vi "Vision_Right_R12.vi"() -> ()   [LabVIEW 2015]
uses:
  <vilib>/vision/Pattern Matching.llb/IMAQ Curve Parameters.ctl
  <vilib>/vision/Pattern Matching.llb/IMAQ Match Range Setting.ctl
panel:
  out "Tracking Info":T1
  out "dT":u32
  out "Avg Scale":dbl=50.23627395629883
  out "Avg Score":dbl=800.1138671875
  out "Current Search Settings":T4={"Curve Parameters"={"Extraction Mode"=1, "Edge Threshold"=150, "Edge Filter Size"=0, "Min Length"=25, "Row Search Step Size"=15, "Col Search Step Size"=15, "Max Endpoint Gap"=2, "Closed"=TRUE, "Subpixel"=TRUE}, "Match Mode"={"Rotation"=TRUE, "Scale"=TRUE, "Occlusion"=TRUE, "Reserved"=FALSE, "Reserved"=FALSE, "Reserved"=FALSE}, "Range Settings"=[{"Match Constraints"=0, "Min"=-5.0, "Max"=5.0}, {"Match Constraints"=1, "Min"=45.23627395629883, "Max"=55.23627395629883}, {"Match Constraints"=2, "Min"=0.0, "Max"=25.0}], "Number of Matches"=1, "Minimum Match Score"=700.1139, "SubPixel Accuracy"=TRUE, "Adv. Geometric Match Options 2"=[{"Setup Data Item"=20, "Item Value"=0.0}, {"Setup Data Item"=22, "Item Value"=1.0}]} {"Curve Parameters"."Extraction Mode" items=["Normal", "Uniform Regions"]; "Curve Parameters"."Edge Filter Size" items=["Fine", "Normal", "Contour Tracing"]; "Curve Parameters"."Max Endpoint Gap" min=0; "Curve Parameters"."Col Search Step Size" min=1 max=255 step=1; "Curve Parameters"."Row Search Step Size" min=1 max=255 step=1; "Curve Parameters"."Min Length" min=0; "Curve Parameters"."Edge Threshold" min=1 max=350 step=1; "Range Settings"."Max" format="%.2f"; "Range Settings"."Min" format="%.2f"; "Range Settings"."Match Constraints" items=["Rotation Angle (degrees)", "Scale Factor (%)", "Occlusion (%)"]}
  out "Valid Scale History":dbl[](array[numeric])=[50.547454833984375, 50.07851791381836, 50.25061798095703, 50.25061798095703, 50.054161071777344, 50.02944564819336, 50.078575134277344, 50.081233978271484, 50.078975677490234, 50.078575134277344, 50.07851791381836, 50.6029052734375, 50.602447509765625, 50.602447509765625, 50.58179473876953, 51.42407989501953, 50.560218811035156, 51.42409896850586, 0.0, 50.602447509765625] format="%#_13g"
  out "Valid Score History":dbl[](array[numeric])=[802.5203247070312, 804.2725830078125, 794.4934692382812, 794.4934692382812, 804.7894897460938, 809.00341796875, 804.2725830078125, 805.539794921875, 804.2725830078125, 803.1467895507812, 804.2725830078125, 777.2046508789062, 774.6702270507812, 774.6702270507812, 777.9379272460938, 790.3563232421875, 777.9379272460938, 790.3563232421875, 0.0, 777.2046508789062] format="%#_13g"
  out "Valid Beacon History - in":bool[](array[boolean])=[TRUE, TRUE, TRUE, TRUE, TRUE, TRUE, TRUE, TRUE, TRUE, TRUE, TRUE, TRUE, TRUE, TRUE, TRUE, TRUE, TRUE, TRUE, FALSE, TRUE]
  out "Startup Flag":bool
  out "Current Tempalte State":T5(ring)=enum."Short Range"
  out "Lock Status":bool=TRUE
  out "Y Coordinates":sgl[](array[numeric])=[153.02994, 149.48933, 150.4864, 150.33003, 0.0]
  out "X Coordinates":sgl[](array[numeric])=[91.3685, 123.99656, 161.27843, 197.4523, 0.0]
  out "Beacons Found":bool[](array[boolean])=[TRUE, TRUE, TRUE, TRUE, FALSE]
  out "Right Image out":T6(plugin-control)
  in  "Initial State":T5(ring)=enum."Short Range"
  in  "History Size":i32=20
  in  "INITIAL Search Settings":T4={"Curve Parameters"={"Extraction Mode"=1, "Edge Threshold"=150, "Edge Filter Size"=0, "Min Length"=25, "Row Search Step Size"=15, "Col Search Step Size"=15, "Max Endpoint Gap"=2, "Closed"=TRUE, "Subpixel"=TRUE}, "Match Mode"={"Rotation"=TRUE, "Scale"=TRUE, "Occlusion"=TRUE, "Reserved"=FALSE, "Reserved"=FALSE, "Reserved"=FALSE}, "Range Settings"=[{"Match Constraints"=0, "Min"=-5.0, "Max"=5.0}, {"Match Constraints"=1, "Min"=20.0, "Max"=60.0}, {"Match Constraints"=2, "Min"=0.0, "Max"=25.0}], "Number of Matches"=1, "Minimum Match Score"=750.0, "SubPixel Accuracy"=TRUE, "Adv. Geometric Match Options 2"=[{"Setup Data Item"=20, "Item Value"=0.0}, {"Setup Data Item"=22, "Item Value"=1.0}]} {"Curve Parameters"."Extraction Mode" items=["Normal", "Uniform Regions"]; "Curve Parameters"."Edge Filter Size" items=["Fine", "Normal", "Contour Tracing"]; "Curve Parameters"."Max Endpoint Gap" min=0; "Curve Parameters"."Col Search Step Size" min=1 max=255 step=1; "Curve Parameters"."Row Search Step Size" min=1 max=255 step=1; "Curve Parameters"."Min Length" min=0; "Curve Parameters"."Edge Threshold" min=1 max=350 step=1; "Range Settings"."Max" format="%.2f"; "Range Settings"."Min" format="%.2f"; "Range Settings"."Match Constraints" items=["Rotation Angle (degrees)", "Scale Factor (%)", "Occlusion (%)"]; "Adv. Geometric Match Options 2"."Setup Data Item" items=["Curve Extraction Mode", "Curve Edge Threshold", "Curve Edge Filter Size", "Min Curve Length", "Curve Row Search Step Size", "Curve Col Search Step Size", "Curve Max Endpoint Gap", "Extract Closed Curves", "Enable Subpixel Curve Extraction", "Enable Correlation Score", "Enable Subpixel Accuracy", "Subpixel Iterations", "Subpixel Tolerance", "Initial Match List Length", "Enable Target Template Curve Score", "Min Match Separation Distance", "Min Match Separation Angle", "Min Match Separation Scale", "Max Match Overlap", "Enable Coarse Result", "Enable Calibration Support", "Enable Contrast Reversal", "Search Strategy", "Refinement Match Factor", "Subpixel Match Factor"]}
  # "Range"
  # "Range"
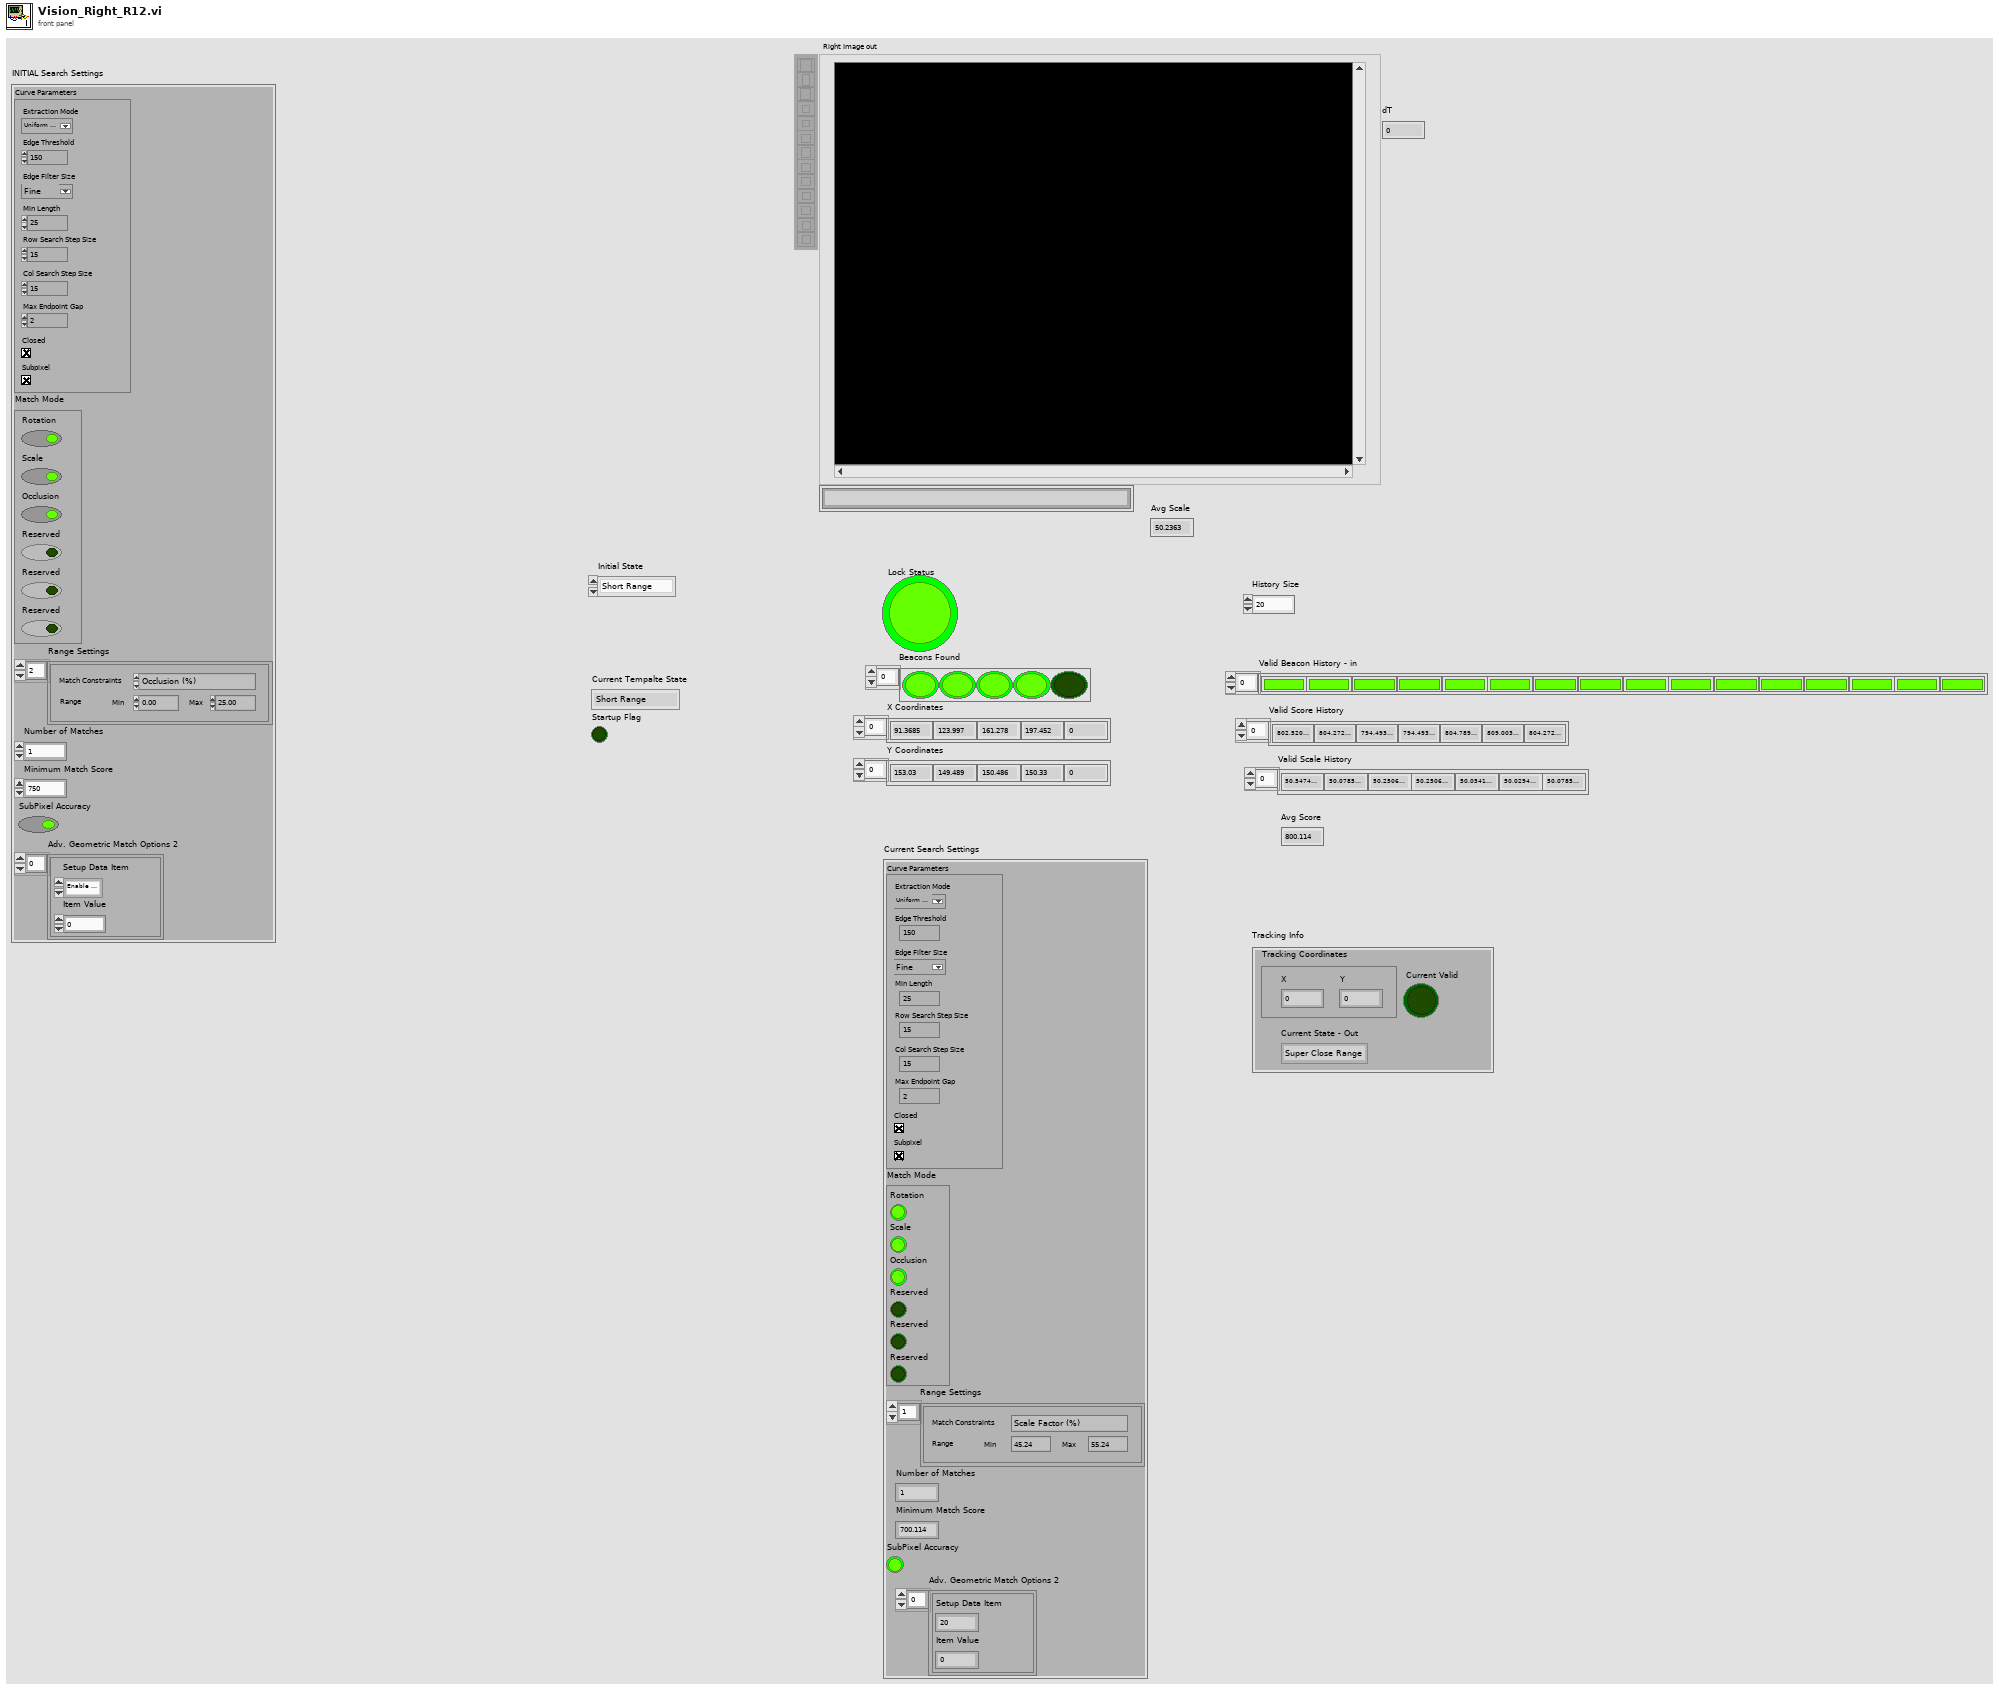
[diagram p1: front panel]
types:
  T1 = cluster{"Tracking Coordinates":cluster{"X":dbl, "Y":dbl}, "Current Valid":bool, "Current State - Out":enum16{"Super Close Range", "Short Range", "Long Range"}}
  T2 = typedef "IMAQ Curve Parameters.ctl" = cluster{"Extraction Mode":u32, "Edge Threshold":i32, "Edge Filter Size":u32, "Min Length":i32, "Row Search Step Size":i32, "Col Search Step Size":i32, "Max Endpoint Gap":i32, "Closed":bool, "Subpixel":bool}
  T3 = typedef "IMAQ Match Range Setting.ctl" = cluster{"Match Constraints":u32, "Min":dbl, "Max":dbl}
  T4 = cluster{"Curve Parameters":T2, "Match Mode":cluster{"Rotation":bool, "Scale":bool, "Occlusion":bool, "Reserved":bool, "Reserved":bool, "Reserved":bool}, "Range Settings":T3[], "Number of Matches":i32, "Minimum Match Score":sgl, "SubPixel Accuracy":bool, "Adv. Geometric Match Options 2":cluster{"Setup Data Item":u16, "Item Value":dbl}[]}
  T5 = enum16{"Super Close Range", "Short Range", "Long Range"}
  T6 = typedef "IMAQ Image.ctl" = refnum<image>
  T7 = typedef "Image Type" = u32
  T8 = typedef "ROI Descriptor" = cluster{"Global Rectangle":i32[], "Contours":cluster{"ID":enum32{"External", "Internal"}, "Type":u32, "Coordinates":i32[]}[]}
  T9 = cluster{"Valid Beacon History\nOut":bool[], "Valid Score History\nOut":dbl[], "Valid Scale History\nOut":dbl[]}
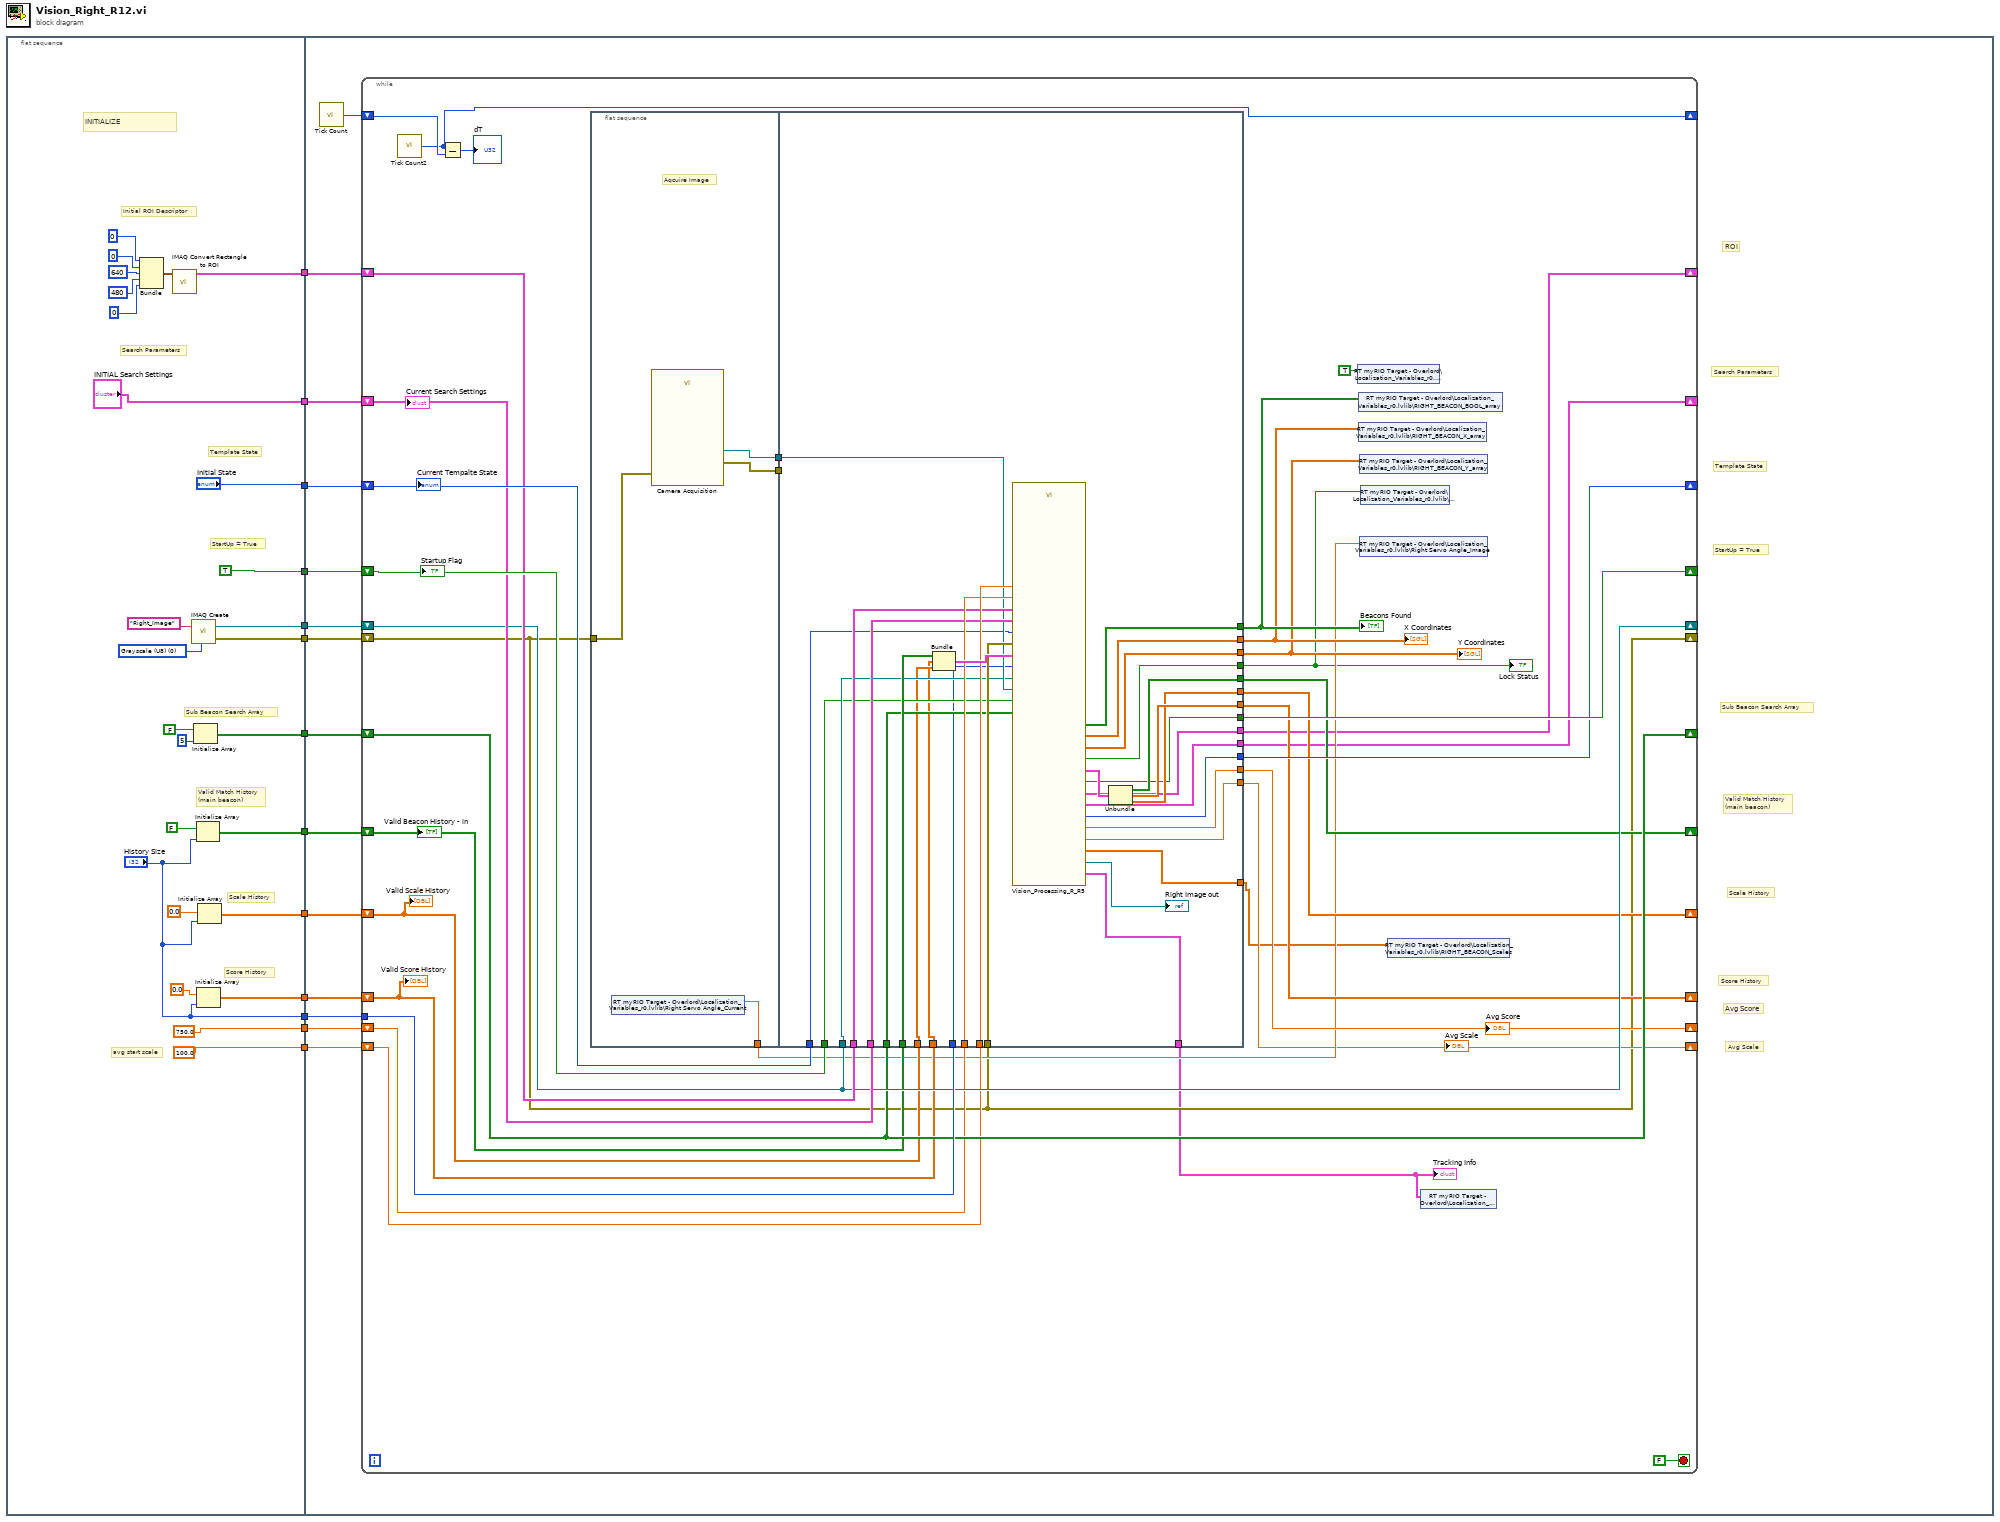
[diagram p0: block diagram]
diagram:
  n1 = flat-sequence {
    tunnel: [w26] -> w13
    tunnel: ["INITIAL Search Settings"] -> w12
    tunnel: ["Initial State"] -> w11
    tunnel: [TRUE] -> w10
    tunnel: [w23] -> w9
    tunnel: [w22] -> w8
    tunnel: [w21] -> w7
    tunnel: [w20] -> w6
    tunnel: [w19] -> w5
    tunnel: [w18] -> w4
    tunnel: ["History Size"] -> w3
    tunnel: [750.0] -> w2
    tunnel: [100.0] -> w1
    tunnel: w13 -> [w53]
    tunnel: w12 -> [w52]
    tunnel: w11 -> [w51]
    tunnel: w10 -> [w50]
    tunnel: w9 -> [w45]
    tunnel: w8 -> [w44]
    tunnel: w7 -> [w49]
    tunnel: w6 -> [w48]
    tunnel: w5 -> [w47]
    tunnel: w4 -> [w46]
    tunnel: w3 -> [w43]
    tunnel: w2 -> [w42]
    tunnel: w1 -> [w41]
    frame #0 {
      w33 = T7 0 items=["Grayscale (U8)", "Grayscale (I16)", "Grayscale (SGL)", "Complex (CSG)", "RGB (U32)", "HSL (U32)", "RGB (U64)", "Grayscale (U16)"] ("Image Type")
      # "avg start scale"
      # "Score History"
      # "Scale History"
      # "Valid Match History\n(main beacon)"
      # "Sub Beacon Search Array"
      # "Template State"
      # "Search Parameters"
      # "StartUp = True"
      # "Initial ROI Descriptor"
      # "INITIALIZE"
      n2 = Bundle(0, 0, 640, 480, 0) -> (w32:cluster{i32, i32, i32, i32, i32})  [unwired: 1 in]
      n3 = call "IMAQ Convert Rectangle to ROI"("Rectangle"=w32) -> ("ROI Descriptor"=w26:T8)  [unwired: 8 in, 1 out]
      n4 = call "IMAQ Create"("Image Name"="Right_Image", "Image Type"=w33) -> ("New Image"=w23:T6, "error out"=w22:errorcluster)  [unwired: 3 in]
      n5 = Initialize Array(FALSE, 5 ("dimension size")) -> (w21:bool[])
      n6 = Initialize Array(FALSE, "History Size") -> (w20:bool[])
      n7 = Initialize Array(0.0, "History Size") -> (w18:dbl[])
      n8 = Initialize Array(0.0, "History Size") -> (w19:dbl[])
    }
    frame #1 {
      # "Avg Scale"
      # "Avg Score"
      # "Score History"
      # "Scale History"
      # "Valid Match History\n(main beacon)"
      # "Sub Beacon Search Array"
      # "StartUp = True"
      # "Template State"
      # "Search Parameters"
      # "ROI"
      n9 = call "Tick Count"() -> ("Tick Count(mSec)"=w40:u32)
      n10 = while {
        shift-right: [w60] -> _
        shift-left: w53 -> [w84]
        shift-right: [w59] -> _
        shift-left: w52 -> [w83]
        shift-right: [w79] -> _
        shift-left: w51 -> [w87]
        shift-right: [w80] -> _
        shift-left: w50 -> [w85]
        shift-right: [w78] -> _
        shift-left: w49 -> [w78]
        shift-right: [w77] -> _
        shift-left: w48 -> [w74]
        shift-right: [w76] -> _
        shift-left: w47 -> [w73]
        shift-right: [w75] -> _
        shift-left: w46 -> [w72]
        shift-right: [w81] -> _
        shift-left: w45 -> [w81]
        shift-right: [w61] -> _
        shift-left: w44 -> [w61]
        tunnel: w43 -> [w82]
        shift-right: [w71] -> _
        shift-left: w42 -> [w70]
        shift-right: [w62] -> _
        shift-left: w41 -> [w69]
        shift-right: [w57] -> _
        shift-left: w40 -> [w58]
        stop <- FALSE stop-if-true
        n11 = call "Tick Count2"() -> ("Tick Count(mSec)"=w57:u32)
        n12 = Subtract(x=w57, y=w58) -> (x-y=→"dT":u32)
        n13 = flat-sequence {
          tunnel: w61 -> [w93]
          tunnel: [w92] -> w88
          tunnel: [w91] -> w86
          tunnel: [w90] -> w64
          tunnel: w88 -> [w117]
          tunnel: w87 -> [w114]
          tunnel: w86 -> [_]
          tunnel: w85 -> [w115]
          tunnel: w81 -> [w116]
          tunnel: w84 -> [w122]
          tunnel: w83 -> [w121]
          tunnel: w78 -> [w118]
          tunnel: w74 -> [w120]
          tunnel: w73 -> [w97]
          tunnel: w72 -> [w96]
          tunnel: w82 -> [w113]
          tunnel: w70 -> [w123]
          tunnel: [w110] -> w67
          tunnel: [w109] -> w66
          tunnel: [w108] -> w65
          tunnel: [w107] -> w63
          tunnel: [w106] -> w77
          tunnel: [w104] -> w76
          tunnel: [w105] -> w75
          tunnel: [w102] -> w80
          tunnel: [w103] -> w60
          tunnel: [w101] -> w59
          tunnel: [w100] -> w79
          tunnel: [w99] -> w71
          tunnel: [w98] -> w62
          tunnel: w69 -> [w124]
          tunnel: w61 -> [w119]
          tunnel: [w95] -> w55
          tunnel: [w94] -> w54
          frame #0 {
            # "Aqcuire Image"
            n14 = shared-variable "RT myRIO Target - Overlord\\Localization_Variables_r0.lvlib\\Right Servo Angle_Current"() -> (w90:dbl)  [unwired: 1 in, 1 out]
            n15 = call "Camera Acquisition"("error in"=w93) -> ("Image Out"=w92:T6, "error out"=w91:errorcluster)  [unwired: 24 in, 1 out]
          }
          frame #1 {
            n16 = Bundle(w120, w96, w97) -> (w125:cluster{bool[], dbl[], dbl[]})  [unwired: 1 in]
            n17 = call "Vision_Processing_R_R5.vi"("Current State"=w114, "Image Dst"=w116, "Inpute Image"=w117, "Startup Flag"=w115, "Current ROI Descriptor"=w122, "Avg Score - Last"=w123, "error in (no error)"=w119, "Current Settings"=w121, "Sub Beacon Search Enable"=w118, "History Data - IN"=w125, "Avg Scale - Last"=w124, "History Size"=w113) -> ("Avg Scale"=w98:dbl, "Avg Score"=w99:dbl, "Tracking Info"=w94:T1, "Next Main ROI Descriptor"=w103:T8, "Beacon - Scales"=w95:sgl[], "History Data - Out"=w112:T9, "Y Coordinates"=w108:sgl[], "Beacons Found"=w110:bool[], "X Coordinates"=w109:sgl[], "Lock Status"=w107:bool, "Startup Flag - out"=w102:bool, "New Settings"=w101:T4, "Next State"=w100:T5, "Right Image 2"=→"Right Image out":T6)  [unwired: 2 in]
            n18 = Unbundle(w112) -> ("Valid Beacon History\nOut"=w106:bool[], "Valid Score History\nOut"=w105:dbl[], "Valid Scale History\nOut"=w104:dbl[])
          }
        }
        n19 = shared-variable "RT myRIO Target - Overlord\\Localization_Variables_r0.lvlib\\RIGHT_FLAG"(TRUE ("RIGHT_FLAG")) -> ()  [unwired: 1 in, 1 out]
        n20 = shared-variable "RT myRIO Target - Overlord\\Localization_Variables_r0.lvlib\\RIGHT_BEACON_BOOL_array"(w67) -> ()  [unwired: 1 in, 1 out]
        n21 = shared-variable "RT myRIO Target - Overlord\\Localization_Variables_r0.lvlib\\RIGHT_BEACON_X_array"(w66) -> ()  [unwired: 1 in, 1 out]
        n22 = shared-variable "RT myRIO Target - Overlord\\Localization_Variables_r0.lvlib\\RIGHT_BEACON_Y_array"(w65) -> ()  [unwired: 1 in, 1 out]
        n23 = shared-variable "RT myRIO Target - Overlord\\Localization_Variables_r0.lvlib\\Right Servo Angle_Image"(w64) -> ()  [unwired: 1 in, 1 out]
        n24 = shared-variable "RT myRIO Target - Overlord\\Localization_Variables_r0.lvlib\\Image Lock - R"(w63) -> ()  [unwired: 1 in, 1 out]
        n25 = shared-variable "RT myRIO Target - Overlord\\Localization_Variables_r0.lvlib\\RIGHT_BEACON_Scales"(w55) -> ()  [unwired: 1 in, 1 out]
        n26 = shared-variable "RT myRIO Target - Overlord\\Localization_Variables_r0.lvlib\\Info - Right"(w54) -> ()  [unwired: 1 in, 1 out]
        "Beacons Found" <- w67
        "X Coordinates" <- w66
        "Y Coordinates" <- w65
        "Lock Status" <- w63
        "Current Tempalte State" <- w87
        "Startup Flag" <- w85
        "Valid Scale History" <- w73
        "Valid Beacon History - in" <- w74
        "Valid Score History" <- w72
        "Current Search Settings" <- w83
        "Avg Score" <- w71
        "Avg Scale" <- w62
        "Tracking Info" <- w54
      }
    }
  }
